vi "Linker.vi"() -> ()   [LabVIEW 2011, in "Messenging.lvlib" / "LinkedEventMessenger.lvclass"]
uses:
  LinkedEventMessenger.lvclass
  Messenger (Parent)/MGR.lvclass
  Receiver/MGR (Receive type).lvclass
panel:
  out "error out":errorcluster
  in  "Outgoing":refnum<class "MGR.lvclass">
  in  "Incoming":refnum<class "MGR (Receive type).lvclass">
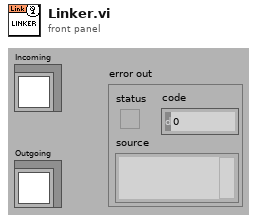
[diagram p1: front panel]
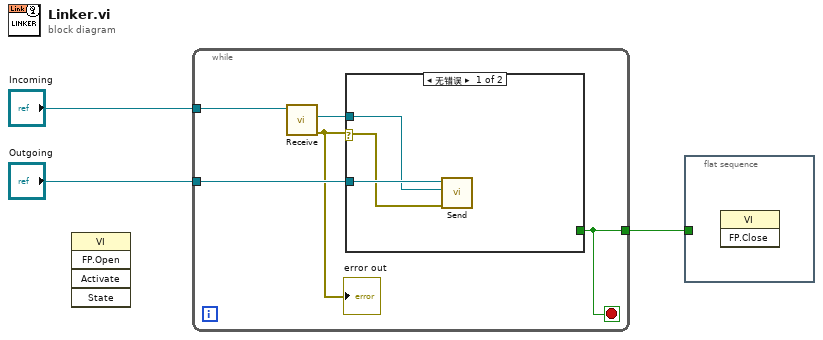
[diagram p0: block diagram]
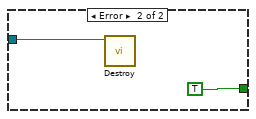
[diagram p2: hidden frame]
diagram:
  n1 = invoke class="VI" method="FP.Open"() -> ()  [unwired: 5 in, 5 out]
  n2 = while {
    tunnel: "Incoming" -> [w8]
    tunnel: "Outgoing" -> [w7]
    tunnel: [w4] -> w1
    stop <- w4 stop-if-true
    n3 = call-dynamic "Receive.vi"("Messenger in"=w8) -> ("error out"=w6:errorcluster, "Message"=w5:refnum<class "MSG.lvclass">)  [unwired: 2 in, 7 out]
    "error out" <- w6
    n4 = case shown="无错误" w6 {
      selector: w6 -> [w9 _]
      tunnel: w7 -> [w11 w13]
      tunnel: w5 -> [w10 _]
      tunnel: [_ TRUE] -> w4
      frame No Error {
        n5 = call-dynamic "Send.vi"("error in (no error)"=w9, "Message"=w10, "MSR Parent in"=w11) -> ()  [unwired: 9 out]
      }
      frame Error {
        n6 = call-dynamic "Destroy.vi"("Messenger in"=w13) -> ()  [unwired: 1 in, 10 out]
      }
    }
  }
  n7 = flat-sequence {
    tunnel: w1 -> [_]
    frame #0 {
      n8 = invoke class="VI" method="FP.Close"() -> ()  [unwired: 3 in, 3 out]
    }
  }
